vi "Measurement Logic.vi"(8 "error in":errorcluster, 9 "measurement configuration":T3={"INTERFACE NAME CAN"="Lorem ipsum dolor sit", "IO Mode CAN"=enum."CAN FD", "FD ISO Mode CAN"=enum."Non-ISO", "Termination CAN"=TRUE, "Baudrate CAN"=64, "FD Baudrate CAN"=64, "INTERFACE NAME LIN"="", "Termination LIN"=TRUE, "CAN interface"="", "LIN interface"="", "Network"="", "DLC INDICATOR"=0, "PAYLOAD INDICATOR"=[0, 0, 0, 0, 0, 0, 0, 0, 0, 0, 0, 0, 0, 0, 0, 0, 0, 0, 0, 0, 0, 0, 0, 0, 0, 0, 0, 0, 0, 0, 0, 0, 0, 0, 0, 0, 0, 0, 0, 0, 0, 0, 0, 0, 0, 0, 0, 0, 0, 0, 0, 0, 0, 0, 0, 0, 0, 0, 0, 0, 0, 0, 0, 0], "IDENTIFIER INDICATOR"=0, "TYPE INDICATOR"=0, "Baudrate LIN"=0} {"Baudrate LIN" format="%x"; "TYPE INDICATOR" items=["CAN Data"=0, "CAN Remote"=1, "CAN Bus Error"=2, "CAN 2.0 Data"=8, "CAN FD Data"=16, "CAN FD+BRS Data"=24, "J1939 Data"=192, "Delay"=224, "Log Trigger"=225, "Start Trigger"=226]; "IDENTIFIER INDICATOR" format="%x"; "PAYLOAD INDICATOR" format="%x"; "Baudrate CAN" format="%x"}, 10 "measure call context in":refnum<class "Measure Call Context.lvclass">, 11 "Stop OOB Server UE":refnum<user-event>) -> (0 "error out":errorcluster, 1 "measurement results":T1 {"Payload LIN" format="%x"; "ID LIN" format="%x"; "Payload CAN" format="%x"; "Type CAN" items=["CAN Data"=0, "CAN Remote"=1, "CAN Bus Error"=2, "CAN 2.0 Data"=8, "CAN FD Data"=16, "CAN FD+BRS Data"=24, "J1939 Data"=192, "Delay"=224, "Log Trigger"=225, "Start Trigger"=226]; "ID CAN" format="%x"}, 2 "measure call context out":refnum<class "Measure Call Context.lvclass">)   [LabVIEW 2025, in "CAN-LIN Frame Generator.lvclass"]
doc: "Contains the core logic for executing the measurement."
uses:
  CAN-LIN Frame Generator.lvclass
  Measurement Configuration.ctl
  CAN-LIN Frame Generator UI/Toggle.ctl
  CAN-LIN Frame Generator UI/XNET Frame Type CAN.ctl
  Measurement Results.ctl
  <vilib>/Plug-In SDKs/Measurements/Measure Call Context/Measure Call Context.lvclass
  XNET Write (Frame CAN).vi
  <vilib>/xnet/xnet.llb/XNET Write (Frame LIN).vi
  CAN-LIN Frame Generator.lvclass/CAN-LIN Frame Generator.ctl
  OOB Data Transfer/OOB Data Transfer.lvlib
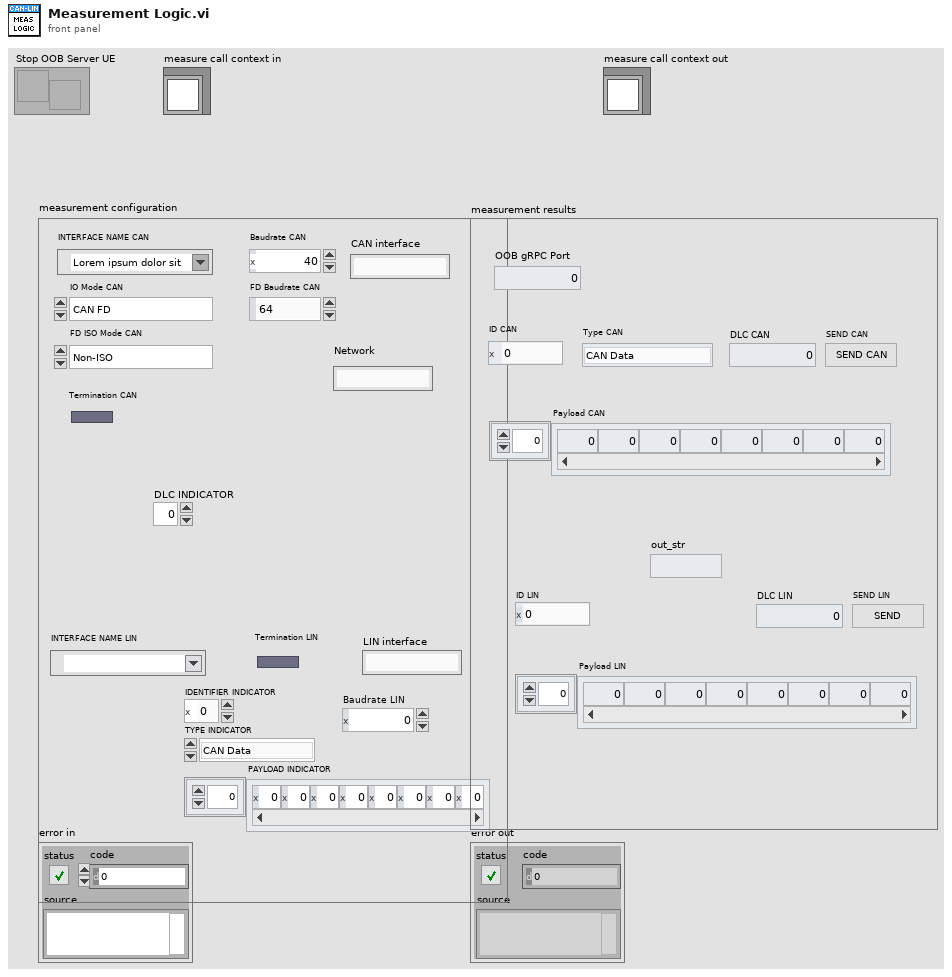
[diagram p1: front panel]
types:
  T1 = typedef "CAN-LIN Frame Generator.lvclass/Measurement Results.ctl" = cluster{"OOB gRPC Port":i32, "ID CAN":u32, "Type CAN":T2, "DLC CAN":u32, "SEND CAN":bool, "Payload CAN":u32[], "ID LIN":u32, "DLC LIN":u32, "SEND LIN":bool, "Payload LIN":u32[], "out_str":string}
  T2 = typedef "XNET Frame Type CAN.ctl" = u32
  T3 = typedef "CAN-LIN Frame Generator.lvclass/Measurement Configuration.ctl" = cluster{"INTERFACE NAME CAN":refnum<k21>, "IO Mode CAN":enum32{"CAN", "CAN FD", "CAN FD + BRS"}, "FD ISO Mode CAN":enum32{"ISO", "Legacy ISO", "Non-ISO"}, "Termination CAN":T4, "Baudrate CAN":u32, "FD Baudrate CAN":u32, "INTERFACE NAME LIN":refnum<k21>, "Termination LIN":T4, "CAN interface":string, "LIN interface":string, "Network":string, "DLC INDICATOR":u32, "PAYLOAD INDICATOR":u32[], "IDENTIFIER INDICATOR":u32, "TYPE INDICATOR":T2, "Baudrate LIN":u32}
  T4 = typedef "Toggle.ctl" = bool
  T5 = typedef "OOB Data Transfer.lvlib/OOB to Logic Data.ctl" = cluster{"PauseResume":bool, "Export":string, "ID CAN":u32, "Type CAN":T2, "DLC CAN":u32, "SEND CAN":bool, "Payload CAN":u32[], "ID LIN":u32, "DLC LIN":u32, "SEND LIN":bool, "Payload LIN":u32[], "out_str":string}
  T6 = typedef "XNET Frame LIN.ctl" = cluster{"timestamp":timestamp, "payload":u8[], "identifier":u32, "type":T7, "event ID":u8, "event slot?":bool, "echo?":bool}
  T7 = typedef "XNET Frame Type LIN.ctl" = u8
  T8 = typedef "XNET Frame CAN.ctl" = cluster{"timestamp":timestamp, "payload":u8[], "identifier":u32, "type":T2, "extended?":bool, "echo?":bool}
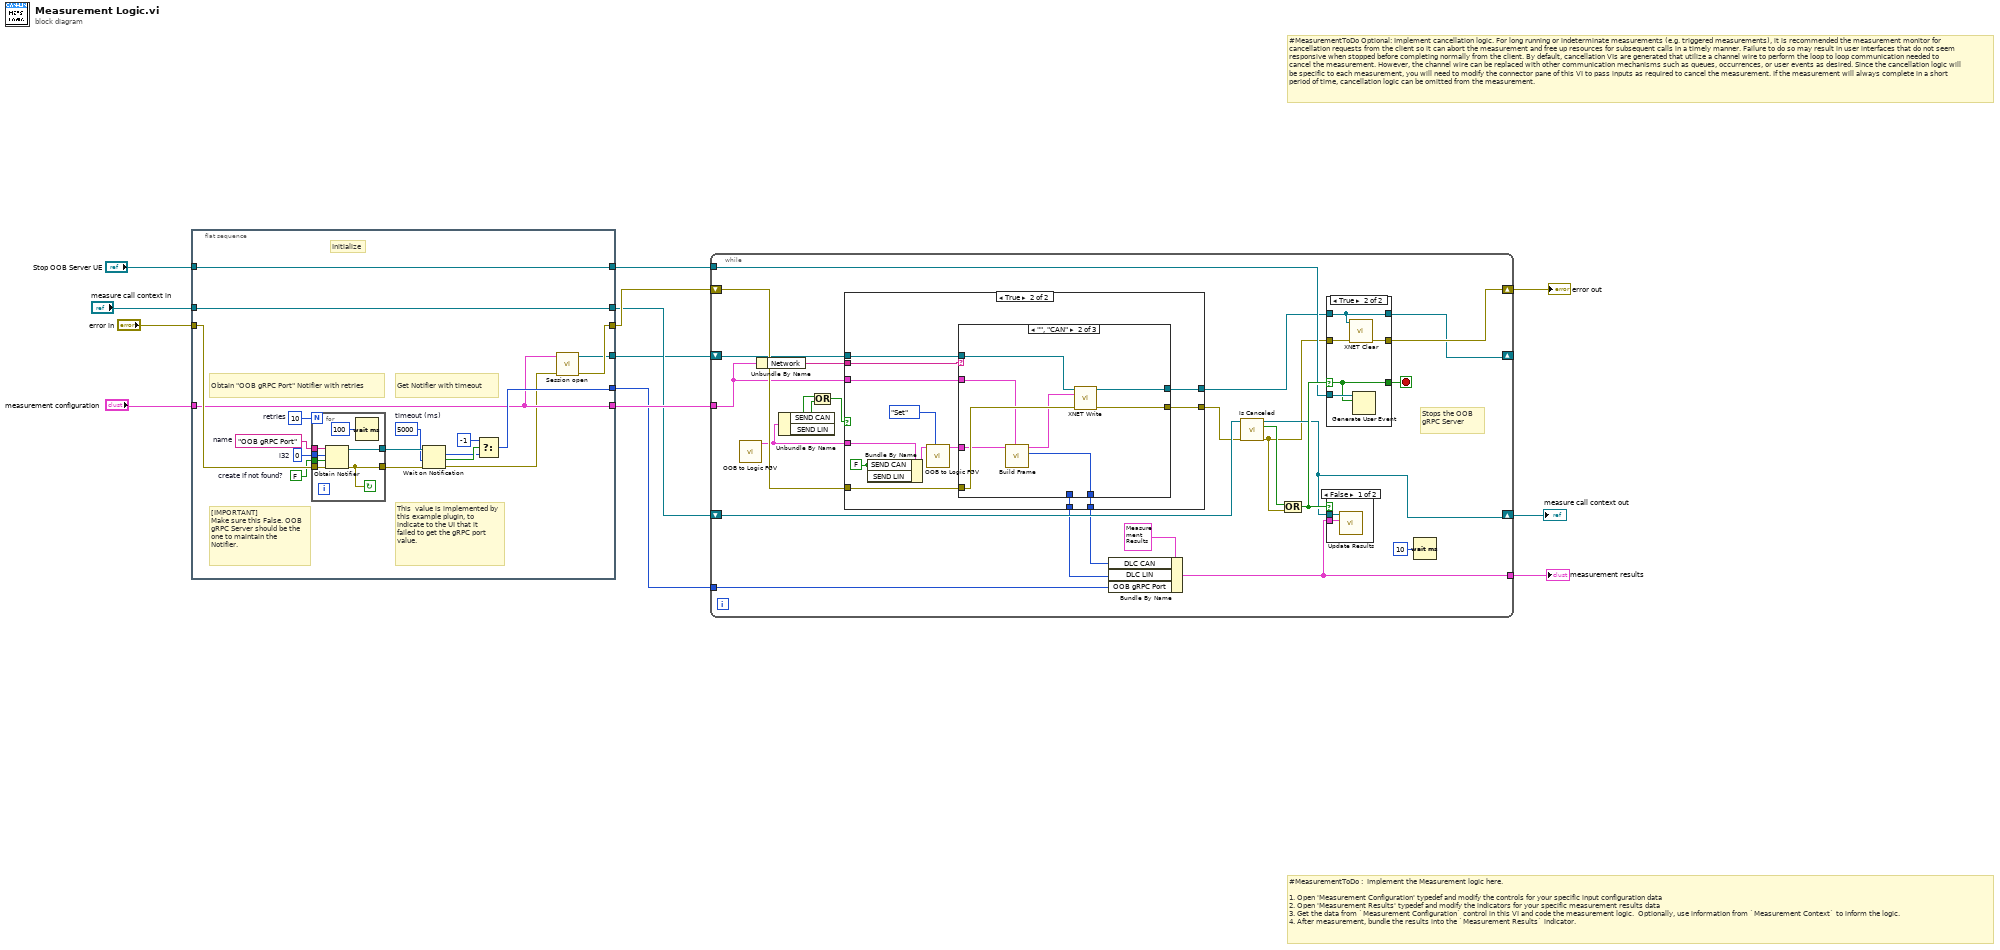
[diagram p0: block diagram]
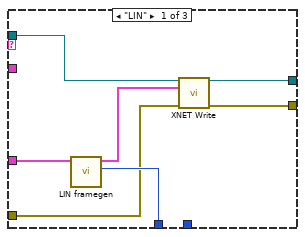
[diagram p3: hidden frame]
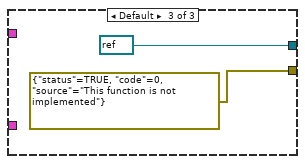
[diagram p4: hidden frame]
diagram:
  # "#MeasurementToDo Optional: Implement cancellation logic. For long running or indeterminate measurements (e.g. triggered measurements), it is recommended the measurement monitor for cancellation requests from the client so it can abort the measurement and free up resources for subsequent calls in a timely manner. Failure to do so may result in user interfaces that do not seem responsive when stopped before completing normally from the client. By default, cancellation VIs are generated that utilize a channel wire to perform the loop to loop communication needed to cancel the measurement. However, the channel wire can be replaced with other communication mechanisms such as queues, occurrences, or user events as desired. Since the cancellation logic will be specific to each measurement, you will need to modify the connector pane of this VI to pass inputs as required to cancel the measurement. If the measurement will always complete in a short period of time, cancellation logic can be omitted from the measurement."
  # "#MeasurementToDo :  Implement the Measurement logic here.\n\n1. Open 'Measurement Configuration' typedef and modify the controls for your specific input configuration data\n2. Open 'Measurement Results' typedef and modify the indicators for your specific measurement results data\n3. Get the data from `Measurement Configuration` control in this VI and code the measurement logic.  Optionally, use information from `Measurement Context` to inform the logic.\n4. After measurement, bundle the results into the `Measurement Results` indicator."
  n1 = flat-sequence {
    tunnel: "error in" -> [w26]
    tunnel: [w15] -> w11
    tunnel: [w24] -> w6
    tunnel: "measurement configuration" -> [w17]
    tunnel: [w17] -> w7
    tunnel: "Stop OOB Server UE" -> [w20]
    tunnel: [w20] -> w5
    tunnel: "measure call context in" -> [w19]
    tunnel: [w19] -> w4
    tunnel: [w14] -> w1
    frame #0 {
      w18 = FALSE  # create if not found?
      w27 = 0  # i32
      w25 = "OOB gRPC Port"  # name
      w28 = 10  # retries
      w29 = 5000  # timeout (ms)
      # "This  value is implemented by this example plugin, to indicate to the UI that it failed to get the gRPC port value."
      # "[IMPORTANT] \nMake sure this False. OOB gRPC Server should be the one to maintain the Notifier."
      # "Initialize"
      # "Obtain \"OOB gRPC Port\" Notifier with retries"
      # "Get Notifier with timeout"
      n2 = for {
        N: w28 -> [_]
        tunnel: [w36] -> w31
        tunnel: [w38] -> w30
        tunnel: w25 -> [w35]
        tunnel: w27 -> [w34]
        tunnel: w26 -> [w33]
        tunnel: w18 -> [w32]
        stop <- w36 continue-if-true
        n3 = Obtain Notifier(name (unnamed)=w35, notification data type=w34, create if not found? (T)=w32, error in (no error)=w33) -> (notifier out=w38:refnum<notifier>, error out=w36:errorcluster)  [unwired: 1 out]
        n4 = Wait (ms)(milliseconds to wait=u32 100) -> ()  [unwired: 1 out]
      }
      n5 = Wait on Notification(notifier=w30, timeout in ms (-1)=w29, error in (no error)=w31) -> (notification=w22:i32, timed out?=w23:bool, error out=w16:errorcluster)  [unwired: 1 in, 1 out]
      n6 = Select(t=-1, s=w23, f=w22) -> (s? t:f=w24:i32)
      n7 = call "Session open.vi"("error in"=w16, "measurement configuration"=w17) -> ("error out"=w15:errorcluster, "session out"=w14:refnum<k21>)  [unwired: 8 in]
    }
  }
  n8 = while {
    tunnel: [w58] -> w13
    tunnel: w7 -> [w42]
    tunnel: w6 -> [w62]
    shift-right: [w52] -> w3
    shift-left: w11 -> [w63]
    tunnel: w5 -> [w59]
    shift-right: [w56] -> w2
    shift-left: w4 -> [w57]
    shift-right: [w50] -> _
    shift-left: w1 -> [w49]
    stop <- w54 stop-if-true
    # "Stops the OOB gRPC Server"
    n9 = call "OOB to Logic FGV.vi"() -> ("OOB to Logic Data out"=w44:T5)  [unwired: 10 in, 1 out]
    n10 = Unbundle By Name(w42) -> ("Network"=w48:string)
    n11 = Unbundle By Name(w44) -> ("SEND CAN"=w40:bool, "SEND LIN"=w39:bool)
    n12 = Or(x=w40, y=w39) -> (x .or. y?=w41:bool)
    n13 = case shown="True" w41 {
      tunnel: w49 -> [w65 w78]
      tunnel: w63 -> [w64 w66]
      tunnel: w48 -> [_ w77]
      tunnel: [w64 w76] -> w55
      tunnel: [w65 w75] -> w51
      tunnel: [_ w74] -> w46
      tunnel: [_ w73] -> w45
      tunnel: w44 -> [_ w72]
      tunnel: w42 -> [_ w68]
      frame False {
      }
      frame True {
        w67 = FALSE ("SEND")
        n14 = Bundle By Name(cluster=w72, "SEND CAN"=w67, "SEND LIN"=w67) -> (w71:T5)
        n15 = call "OOB to Logic FGV.vi"("Op (Get)"=enum16{"Get", "Set"}."Set", "OOB to Logic Data in"=w71) -> ("OOB to Logic Data out"=w69:T5)  [unwired: 8 in, 1 out]
        n16 = case shown="\"\", \"CAN\"" w77 {
          tunnel: w78 -> [w85 w93 _]
          tunnel: w66 -> [w79 w92 _]
          tunnel: [w84 w89 errorcluster {"status"=TRUE, "code"=0, "source"="This function is not implemented"} ("error out")] -> w76
          tunnel: [_ w90 _] -> w74
          tunnel: [w80 _ _] -> w73
          tunnel: [w82 w88 refnum<k21> refnum ("session out")] -> w75
          tunnel: w69 -> [w81 w87 _]
          tunnel: w68 -> [_ w86 _]
          frame "LIN" {
            n17 = call "LIN framegen.vi"("OOB to Logic Data in"=w81) -> ("DLC 2"=w80:u32, "Array"=w83:T6[])  [unwired: 9 in]
            n18 = call-poly "XNET Write.vi"("session in"=w85, "data"=w83, "error in (no error)"=w79) -> ("session out"=w82:refnum<k21>, "error out"=w84:errorcluster)  [unwired: 11 in]
          }
          frame "", "CAN" {
            n19 = call "Build Frame.vi"("measurement configuration"=w86, "OOB to Logic Data in"=w87) -> ("DLC out"=w90:u32, "Array"=w91:T8[])  [unwired: 8 in]
            n20 = call-poly "XNET Write.vi"("session in"=w93, "data"=w91, "error in (no error)"=w92) -> ("session out"=w88:refnum<k21>, "error out"=w89:errorcluster)  [unwired: 11 in]
          }
          frame Default {
          }
        }
      }
    }
    n21 = Bundle By Name(cluster=T1 {"OOB gRPC Port"=0, "ID CAN"=0, "Type CAN"=0, "DLC CAN"=0, "SEND CAN"=FALSE, "Payload CAN"=[0, 0, 0, 0, 0, 0, 0, 0, 0, 0, 0, 0, 0, 0, 0, 0, 0, 0, 0, 0, 0, 0, 0, 0, 0, 0, 0, 0, 0, 0, 0, 0, 0, 0, 0, 0, 0, 0, 0, 0, 0, 0, 0, 0, 0, 0, 0, 0, 0, 0, 0, 0, 0, 0, 0, 0, 0, 0, 0, 0, 0, 0, 0, 0], "ID LIN"=0, "DLC LIN"=0, "SEND LIN"=FALSE, "Payload LIN"=[0, 0, 0, 0, 0, 0, 0, 0], "out_str"=""} ("Measurement Results"), "DLC CAN"=w46, "DLC LIN"=w45, "OOB gRPC Port"=w62) -> (w58:T1)
    n22 = call <vilib>:"Is Canceled.vi"("error in"=w55, "measure call context in"=w57) -> ("error out"=w53:errorcluster, "is canceled?"=w61:bool, "measure call context out"=w56:refnum<class "Measure Call Context.lvclass">)  [unwired: 7 in]
    n23 = Compound Arithmetic op=OR(w61, w53) -> (w60:bool)
    n24 = case shown="True" w60 {
      selector: w60 -> [w98 w102]
      tunnel: w59 -> [_ w103]
      tunnel: [w98 w102] -> w54
      tunnel: w53 -> [w97 w101]
      tunnel: [w97 w100] -> w52
      tunnel: w51 -> [w96 w99]
      tunnel: [w96 w99] -> w50
      frame False {
      }
      frame True {
        n25 = call <vilib>:"XNET Clear.vi"("session in"=w99, "error in (no error)"=w101) -> ("error out"=w100:errorcluster)  [unwired: 13 in]
        n26 = Generate User Event(user event=w103, event data cluster=w102) -> ()  [unwired: 2 in, 2 out]
      }
    }
    n27 = case shown="False" w60 {
      tunnel: w56 -> [w105 _]
      tunnel: w58 -> [w104 _]
      frame False {
        n28 = call <vilib>:"Update Results.vi"("measurement results"=w104, "measure call context in"=w105) -> ()  [unwired: 8 in, 2 out]
      }
      frame True {
      }
    }
    n29 = Wait (ms)(milliseconds to wait=u32 10) -> ()  [unwired: 1 out]
  }
  "error out" <- w3
  "measurement results" <- w13
  "measure call context out" <- w2
